vi "parse_finish_batch_response.vi"(8 "error_in":errorcluster, 11 "SQL_result":variant) -> (0 "error_out":errorcluster)   [LabVIEW 2019]
uses:
  _misc/AULocalize/SubVIs/Get Localized Phrase Compact Interface 0D.vi
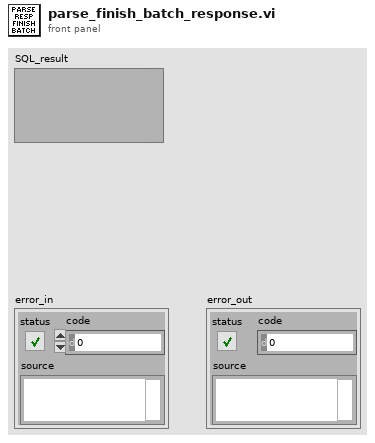
[diagram p1: front panel]
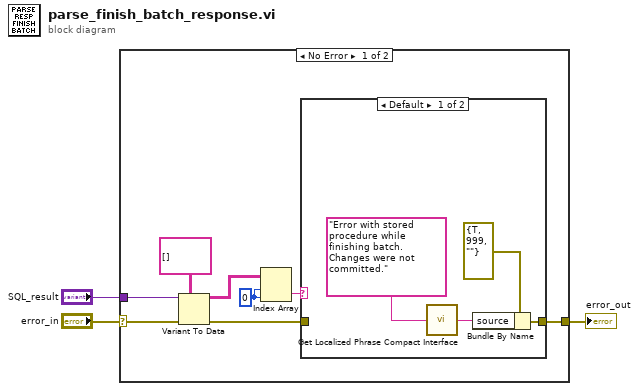
[diagram p0: block diagram]
diagram:
  n1 = case shown="No Error" "error_in" {
    selector: "error_in" -> [w9 w17]
    tunnel: "SQL_result" -> [w10 _]
    tunnel: [w5 w17] -> w1
    frame No Error {
      w4 = 0 ("disabled index (col)")
      n2 = Variant To Data(error in=w9, type=string[][] [], Variant=w10) -> (data=w7:string[][], error out=w6:errorcluster)
      n3 = Index Array(array=w7, index (row)=w4, index (col)=w4) -> (element=w11:string)
      n4 = case shown="Default" w11 {
        tunnel: w6 -> [_ w16]
        tunnel: [w15 w16] -> w5
        frame Default {
          n5 = call-poly "Get Localized Phrase Compact Interface.vi"("Key"="Error with stored procedure while finishing batch. Changes were not committed." ("source")) -> ("Translated Phrase"=w12:string)
          n6 = Bundle By Name(cluster=errorcluster {"status"=TRUE, "code"=999, "source"=""} ("error out"), "source"=w12) -> (w15:errorcluster)
        }
        frame "1" {
        }
      }
    }
    frame Error {
    }
  }
  "error_out" <- w1
